vi "Get Image Information Content.vi"(8 "error in (no error)":errorcluster, 11 "Image":T1) -> (0 "error out":errorcluster, 3 "contrast":sgl)   [LabVIEW 2012]
uses:
  <vilib>/vision/Image Controls.llb/IMAQ Image.ctl
  <vilib>/Analysis/baseanly.llb/Mean (DBL).vi
  <vilib>/gmath/NI_Gmath.lvlib
  <vilib>/Analysis/NI_AALBase.lvlib
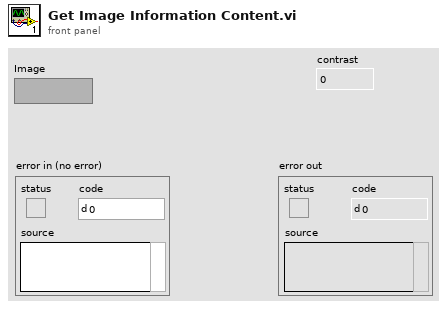
[diagram p1: front panel]
types:
  T1 = typedef "IMAQ Image.ctl" = refnum<image>
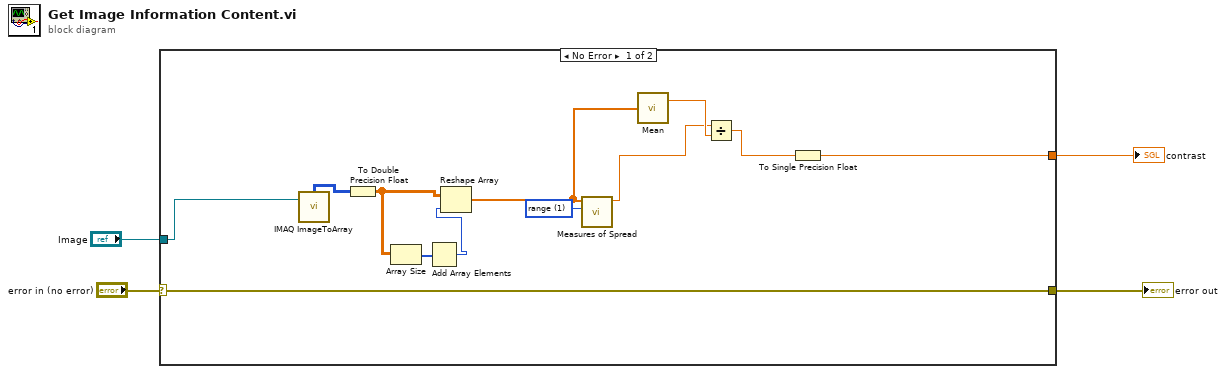
[diagram p0: block diagram]
diagram:
  n1 = case shown="No Error" "error in (no error)" {
    selector: "error in (no error)" -> [w16 w17]
    tunnel: "Image" -> [w9 _]
    tunnel: [w16 w17] -> w2
    tunnel: [w10 _] -> w1
    frame No Error {
      w11 = 1 items=["standard deviation", "range", "mean absolute deviation", "interquartile range"] ("type")
      n2 = call "IMAQ ImageToArray"("Image"=w9) -> ("Image Pixels (U8)"=w15:u8[][])  [unwired: 3 in, 4 out]
      n3 = To Double Precision Float(number=w15) -> (double precision float=w13:dbl[][])
      n4 = Array Size(array=w13) -> (size(s)=w14:i32[])
      n5 = Add Array Elements(numeric array=w14) -> (sum=w12:i32)
      n6 = Reshape Array(w13, w12) -> (w8:dbl[])
      n7 = call <vilib>:"Measures of Spread.vi"("type"=w11, "x array"=w8) -> ("spread value"=w6:dbl)  [unwired: 8 in, 1 out]
      n8 = call-poly <vilib>:"Mean.vi"("X"=w8) -> ("mean"=w7:dbl)  [unwired: 1 out]
      n9 = Divide(x=w6, y=w7) -> (x/y=w5:dbl)
      n10 = To Single Precision Float(number=w5) -> (single precision float=w10:sgl)
    }
    frame Error {
    }
  }
  "contrast" <- w1
  "error out" <- w2
